vi "Test 5.vi"   [LabVIEW 2019]
uses:
  736e36ca-d201-4d61-9dd7-5a8a903a9ac7.vi
  93e37c24-2d72-4c01-aa2a-8225d79ad540.vi
  72ed2c75-68c4-45e6-ba3e-41cefe347f87.vi
  693f8a1d-de51-4b8c-8bcf-b77a035d2a8f.vi
  a161344a-f248-468e-9dcd-b0a79b2b4423.vi
  c835b835-85d9-485c-beb9-6dad4800e08b.vi
  0bc66654-a031-439f-820c-4f9f6562624d.vi
  9e1c42d0-7a69-45bb-9233-67ee3882a033.vi
  867fd164-5876-459f-aa26-76b88d3fff51.vi
  f4de4dee-bbb8-4619-98a2-8609a1925060.vi
  23777dd4-8f3e-4622-9a12-977da9978d21.vi
  edc6580e-75ca-4f12-8ff3-1c8d7cd651f7.vi
  b3638202-8706-45cb-b35d-c907e9c97368.vi
  1e3a4257-6581-4835-b37e-784177fa2f12.vi
  3ff988ee-4feb-49b0-868e-4507fb3a9c7a.vi
  bfd8ad2f-59da-4c70-98bc-ee29fe1e2418.vi
  b7db71a4-6e19-4dbc-bf74-f71ed52b7837.vi
  c30927ab-c643-4aef-8bfa-0f59cb65a99e.vi
  973dfdf0-8b25-4d7d-81a4-c88e7e5a29c4.vi
  13c4d325-1870-4f67-ab67-c133be62a579.vi
  13dea9c8-f20d-4d3b-8f9b-19a6026f4664.vi
  cf393f28-305a-4cae-83a0-a6150f14f9fc.vi
  331a9b46-34b8-4f0c-a9f7-00be6b539627.vi
  f9f875b0-e25d-4d7f-affc-feba7799ba7f.vi
  2297401b-a350-41c4-ae32-f5d0f094e5b4.vi
  a2ca14b0-8187-4a74-bfed-b9dbce034087.vi
  1ec20754-382b-4294-b03e-c13ac0bfef72.vi
  891d9368-8b57-47b4-add5-d0876c7a6189.vi
  0e0f6057-31ed-4d98-a48c-2d8118134b46.vi
  789ab5ea-a867-43ec-b3ec-5bbdc7add248.vi
  b4aade01-484d-45fe-bd25-7c6c7aa8faa7.vi
  b59d95f6-e603-40ea-bc94-15ae8e49d51b.vi
  46ff5037-6347-443d-8af4-35d75e4d7e57.vi
  e9658c67-b325-4e8f-872c-0a8a354b9d3e.vi
  77965676-ca86-458a-870c-14509e410812.vi
  b407d156-6ecf-4492-b562-aa514cd40f4d.vi
  3e3be035-03d0-41f0-b51c-020110ff66b2.vi
  659b2b82-5198-4498-9da7-c3aea3f183cf.vi
  80f0d3fd-3640-4e05-a816-be2c6300e104.vi
  7563cd81-9796-47cf-bc42-87963b6b8f6b.vi
  736e36ca-d201-4d61-9dd7-5a8a903a9ac7.vi/c02bd788-a678-474c-a0c0-234b747aa70c.vi
  693f8a1d-de51-4b8c-8bcf-b77a035d2a8f.vi/a92767fe-f7a6-435d-8353-8231f8cd058c.vi
  693f8a1d-de51-4b8c-8bcf-b77a035d2a8f.vi/21b8ebf0-c13d-419e-82c2-b417d56f3ba1.vi
  a161344a-f248-468e-9dcd-b0a79b2b4423.vi/e43970a7-4556-48ad-ab99-b11f8bbc4b4b.vi
  c835b835-85d9-485c-beb9-6dad4800e08b.vi/30e9680b-6254-404d-a149-a79a1f193854.vi
  867fd164-5876-459f-aa26-76b88d3fff51.vi/099503f4-cda3-4fe7-b577-d7c31d643920.vi
  f4de4dee-bbb8-4619-98a2-8609a1925060.vi/4690f123-cc7b-49a7-8c41-9268aca51ebb.vi
  23777dd4-8f3e-4622-9a12-977da9978d21.vi/5aa92e07-19a0-4715-b2a4-bd2183a10b00.vi
  3ff988ee-4feb-49b0-868e-4507fb3a9c7a.vi/327e55ad-4f13-4f1d-9e58-d5b90e2a486a.vi
  bfd8ad2f-59da-4c70-98bc-ee29fe1e2418.vi/db60f5a0-9537-4c7e-b802-706ccbc92b29.vi
  973dfdf0-8b25-4d7d-81a4-c88e7e5a29c4.vi/92006720-ad0b-467a-b6cb-cc152e365a30.vi
  13c4d325-1870-4f67-ab67-c133be62a579.vi/b8b32592-efa2-4b69-aac0-9d59bb8023b6.vi
  0e0f6057-31ed-4d98-a48c-2d8118134b46.vi/2b744327-1f11-4acc-9221-9a9ba12e084f.vi
  3e3be035-03d0-41f0-b51c-020110ff66b2.vi/d957c6e5-dde0-41c1-9dee-7c1d1782643c.vi
  659b2b82-5198-4498-9da7-c3aea3f183cf.vi/d589f6cf-2ce4-49a5-bd61-ca66bac5b03e.vi
  7563cd81-9796-47cf-bc42-87963b6b8f6b.vi/a0e29051-3a36-415c-b7d2-f8dc20573656.vi
  693f8a1d-de51-4b8c-8bcf-b77a035d2a8f.vi/a92767fe-f7a6-435d-8353-8231f8cd058c.vi/c096529f-17e0-47ad-8482-080bb2ac5765.vi
  693f8a1d-de51-4b8c-8bcf-b77a035d2a8f.vi/a92767fe-f7a6-435d-8353-8231f8cd058c.vi/f51231d8-8f8a-4675-a762-b51b171420a8.vi
  Arrays Library/VIs/Public/Utils/Get Sizes.vi
  Variant Attribute Library/Variant Attributes.lvlib
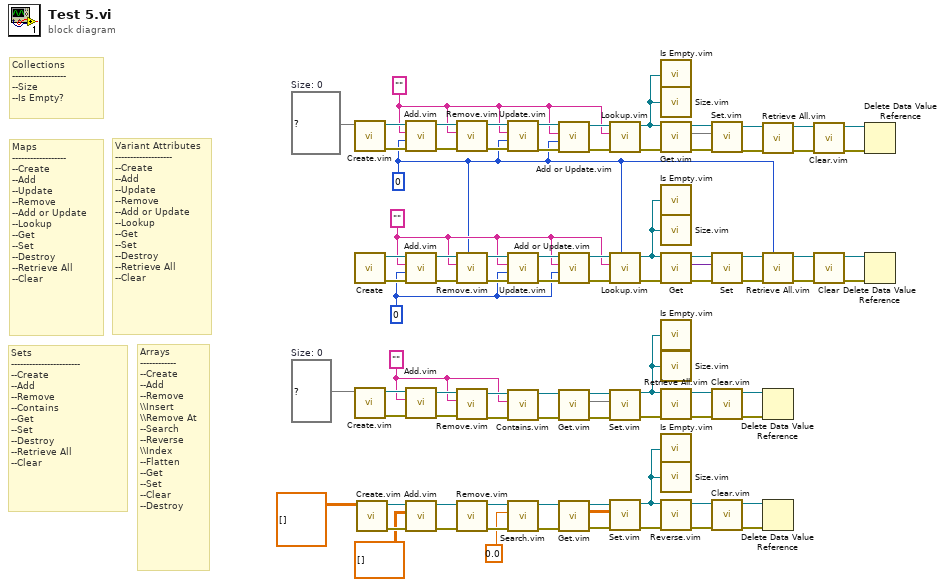
[diagram p0: block diagram]
diagram:
  w7 = ""
  w37 = set{string} {}  # Size: 0
  w55 = 0
  w52 = ""
  w47 = 0
  w69 = ""
  w68 = map{string, i32} {}  # Size: 0
  # "Arrays\n------------\n--Create\n--Add\n--Remove\n\\\\Insert\n\\\\Remove At\n--Search\n--Reverse\n\\\\Index\n--Flatten\n--Get\n--Set\n--Clear\n--Destroy"
  # "Variant Attributes\n-------------------\n--Create\n--Add\n--Update\n--Remove\n--Add or Update\n--Lookup\n--Get\n--Set\n--Destroy\n--Retrieve All\n--Clear"
  # "Sets\n-----------------------\n--Create\n--Add\n--Remove\n--Contains\n--Get\n--Set\n--Destroy\n--Retrieve All\n--Clear"
  # "Collections\n------------------\n--Size\n--Is Empty?"
  # "Maps\n------------------\n--Create\n--Add\n--Update\n--Remove\n--Add or Update\n--Lookup\n--Get\n--Set\n--Destroy\n--Retrieve All\n--Clear"
  n1 = call "Create.vim"("Map"=w68) -> ("error out"=w82:errorcluster, "Map DVR out"=w85:refnum<data-value>)  [unwired: 9 in]
  n2 = call "Create.vi"() -> ("error out"=w66:errorcluster, "Variant DVR out"=w67:refnum<data-value>)  [unwired: 10 in]
  n3 = call "Create.vim"("Set"=w37) -> ("error out"=w40:errorcluster, "Set DVR out"=w41:refnum<data-value>)  [unwired: 9 in]
  n4 = call "Create.vim"("Array"=dbl[][][] [] ("initialized array")) -> ("error out"=w25:errorcluster, "Array DVR out"=w26:refnum<data-value>)  [unwired: 9 in]
  n5 = call "Add.vim"("error in (no error)"=w82, "Value"=w47, "Key"=w69, "Map DVR in"=w85) -> ("error out"=w83:errorcluster, "Map DVR out"=w84:refnum<data-value>)  [unwired: 5 in, 1 out]
  n6 = call "Add.vim"("error in (no error)"=w66, "Value"=w55, "Name"=w52, "Variant DVR in"=w67) -> ("error out"=w60:errorcluster, "Variant DVR out"=w61:refnum<data-value>)  [unwired: 5 in, 1 out]
  n7 = call "Add.vim"("error in (no error)"=w40, "Element"=w7, "Set DVR in"=w41) -> ("error out"=w38:errorcluster, "Set DVR out"=w39:refnum<data-value>)  [unwired: 6 in, 1 out]
  n8 = call "Add.vim"("error in (no error)"=w25, "Element"=dbl[][] [] ("initialized array"), "Array DVR in"=w26) -> ("error out"=w22:errorcluster, "Array DVR out"=w23:refnum<data-value>)  [unwired: 7 in]
  n9 = call "Remove.vim"("error in (no error)"=w83, "Key"=w69, "Map DVR in"=w84) -> ("error out"=w80:errorcluster, "Map DVR out"=w81:refnum<data-value>)  [unwired: 5 in, 2 out]
  n10 = call "Remove.vim"("Type/Default"=w47, "error in (no error)"=w60, "Name"=w52, "Variant DVR in"=w61) -> ("error out"=w58:errorcluster, "Variant DVR out"=w59:refnum<data-value>)  [unwired: 4 in, 2 out]
  n11 = call "Remove.vim"("error in (no error)"=w38, "Element"=w7, "Set DVR in"=w39) -> ("error out"=w35:errorcluster, "Set DVR out"=w36:refnum<data-value>)  [unwired: 6 in, 1 out]
  n12 = call "Remove.vim"("error in (no error)"=w22, "Array DVR in"=w23) -> ("error out"=w19:errorcluster, "Array DVR out"=w20:refnum<data-value>)  [unwired: 7 in, 1 out]
  n13 = call "Update.vim"("error in (no error)"=w80, "Value"=w47, "Key"=w69, "Map DVR in"=w81) -> ("error out"=w79:errorcluster, "Map DVR out"=w78:refnum<data-value>)  [unwired: 5 in, 1 out]
  n14 = call "Update.vim"("error in (no error)"=w58, "Value"=w55, "Name"=w52, "Variant DVR in"=w59) -> ("error out"=w57:errorcluster, "Variant DVR out"=w56:refnum<data-value>)  [unwired: 5 in, 1 out]
  n15 = call "Contains.vim"("error in (no error)"=w35, "Element"=w7, "Set DVR in"=w36) -> ("error out"=w34:errorcluster, "Set DVR out"=w9:refnum<data-value>)  [unwired: 6 in, 1 out]
  n16 = call "Search.vim"("error in (no error)"=w19, "Element"=0.0 ("element"), "Array DVR in"=w20) -> ("error out"=w16:errorcluster, "Array DVR out"=w17:refnum<data-value>)  [unwired: 6 in, 1 out]
  n17 = call "Add or Update.vim"("error in (no error)"=w79, "Value"=w47, "Key"=w69, "Map DVR in"=w78) -> ("error out"=w76:errorcluster, "Map DVR out"=w77:refnum<data-value>)  [unwired: 4 in, 2 out]
  n18 = call "Add or Update.vim"("error in (no error)"=w57, "Value"=w55, "Name"=w52, "Variant DVR in"=w56) -> ("error out"=w53:errorcluster, "Variant DVR out"=w54:refnum<data-value>)  [unwired: 4 in, 2 out]
  n19 = call "Get.vim"("error in (no error)"=w34, "Set DVR in"=w9) -> ("error out"=w32:errorcluster, "Set"=w31:set{string}, "Set DVR out"=w33:refnum<data-value>)  [unwired: 7 in]
  n20 = call "Get.vim"("error in (no error)"=w16, "Array DVR in"=w17) -> ("error out"=w14:errorcluster, "Array"=w13:dbl[][][], "Array DVR out"=w15:refnum<data-value>)  [unwired: 7 in]
  n21 = call "Lookup.vim"("error in (no error)"=w76, "Key"=w69, "Map DVR in"=w77) -> ("error out"=w75:errorcluster, "Map DVR out"=w3:refnum<data-value>)  [unwired: 5 in, 2 out]
  n22 = call "Lookup.vim"("Type/Default"=w47, "error in (no error)"=w53, "Name"=w52, "Variant DVR in"=w54) -> ("error out"=w51:errorcluster, "Variant DVR out"=w4:refnum<data-value>)  [unwired: 4 in, 2 out]
  n23 = call "Set.vim"("error in (no error)"=w32, "Set"=w31, "Set DVR in"=w33) -> ("error out"=w30:errorcluster, "Set DVR out"=w6:refnum<data-value>)  [unwired: 7 in]
  n24 = call "Set.vim"("error in (no error)"=w14, "Array"=w13, "Array DVR in"=w15) -> ("error out"=w12:errorcluster, "Array DVR out"=w5:refnum<data-value>)  [unwired: 7 in]
  n25 = call "Is Empty.vim"("DVR in"=w3) -> ()  [unwired: 4 in, 1 out]
  n26 = call "Size.vim"("DVR in"=w3) -> ()  [unwired: 4 in, 1 out]
  n27 = call "Get.vim"("error in (no error)"=w75, "Map DVR in"=w3) -> ("error out"=w73:errorcluster, "Map"=w70:map{string, i32}, "Map DVR out"=w74:refnum<data-value>)  [unwired: 7 in]
  n28 = call "Is Empty.vim"("DVR in"=w4) -> ()  [unwired: 4 in, 1 out]
  n29 = call "Size.vim"("DVR in"=w4) -> ()  [unwired: 4 in, 1 out]
  n30 = call "Get.vi"("error in (no error)"=w51, "Variant DVR in"=w4) -> ("error out"=w50:errorcluster, "Variant"=w48:variant, "Variant DVR out"=w49:refnum<data-value>)  [unwired: 7 in]
  n31 = call "Is Empty.vim"("DVR in"=w6) -> ()  [unwired: 4 in, 1 out]
  n32 = call "Size.vim"("DVR in"=w6) -> ()  [unwired: 4 in, 1 out]
  n33 = call "Retrieve All.vim"("error in (no error)"=w30, "Set DVR in"=w6) -> ("error out"=w29:errorcluster, "Set DVR out"=w10:refnum<data-value>)  [unwired: 7 in, 1 out]
  n34 = call "Is Empty.vim"("DVR in"=w5) -> ()  [unwired: 4 in, 1 out]
  n35 = call "Size.vim"("DVR in"=w5) -> ()  [unwired: 4 in, 1 out]
  n36 = call "Reverse.vim"("error in (no error)"=w12, "Array DVR in"=w5) -> ("error out"=w11:errorcluster, "Array DVR out"=w8:refnum<data-value>)  [unwired: 8 in]
  n37 = call "Set.vim"("error in (no error)"=w73, "Map"=w70, "Map DVR in"=w74) -> ("error out"=w71:errorcluster, "Map DVR out"=w72:refnum<data-value>)  [unwired: 6 in, 1 out]
  n38 = call "Set.vi"("error in (no error)"=w50, "Variant"=w48, "Variant DVR in"=w49) -> ("error out"=w46:errorcluster, "Variant DVR out"=w86:refnum<data-value>)  [unwired: 6 in, 1 out]
  n39 = call "Clear.vim"("error in (no error)"=w29, "Set DVR in"=w10) -> ("error out"=w27:errorcluster, "Set DVR out"=w28:refnum<data-value>)  [unwired: 8 in]
  n40 = call "Clear.vim"("error in (no error)"=w11, "Array DVR in"=w8) -> ("error out"=w1:errorcluster, "Array DVR out"=w2:refnum<data-value>)  [unwired: 8 in]
  n41 = call "Retrieve All.vim"("error in (no error)"=w71, "Map DVR in"=w72) -> ("error out"=w64:errorcluster, "Map DVR out"=w65:refnum<data-value>)  [unwired: 6 in, 2 out]
  n42 = call "Retrieve All.vim"("Base Type"=w47, "error in (no error)"=w46, "Variant DVR in"=w86) -> ("error out"=w44:errorcluster, "Variant DVR out"=w45:refnum<data-value>)  [unwired: 5 in, 2 out]
  n43 = Delete Data Value Reference(data value reference=w28, error in=w27) -> ()  [unwired: 2 out]
  n44 = Delete Data Value Reference(data value reference=w2, error in=w1) -> ()  [unwired: 2 out]
  n45 = call "Clear.vim"("error in (no error)"=w64, "Map DVR in"=w65) -> ("error out"=w63:errorcluster, "Map DVR out"=w62:refnum<data-value>)  [unwired: 8 in]
  n46 = call "Clear.vi"("error in (no error)"=w44, "Variant DVR in"=w45) -> ("error out"=w42:errorcluster, "Variant DVR out"=w43:refnum<data-value>)  [unwired: 8 in]
  n47 = Delete Data Value Reference(data value reference=w62, error in=w63) -> ()  [unwired: 2 out]
  n48 = Delete Data Value Reference(data value reference=w43, error in=w42) -> ()  [unwired: 2 out]
